vi "new.vi"(7 "waitgroups":refnum<data-value>, 8 "error in (no error)":errorcluster, 11 "max_waitgroup_processes":i32=1) -> (0 "error out":errorcluster, 3 "waitgroup":T1)   [LabVIEW 2015, in "lv-waitgroup.lvlib"]
doc: "new.vi when provided with a valid variant DVR and a set number of max_processes, it will create an ID and generate a \"Waitgroup\" reference, which combines the provided DVR reference with the ID for the waitgroup that can be used for a number of downstream/child functions. This waitgroup reference can be used to group processes under the same waitgroup. Use new.vi every time you want to group processes."
uses:
  lv-waitgroup.lvlib
  _controls/api_waitgroup.ctl
  private/_controls/waitgroup.ctl
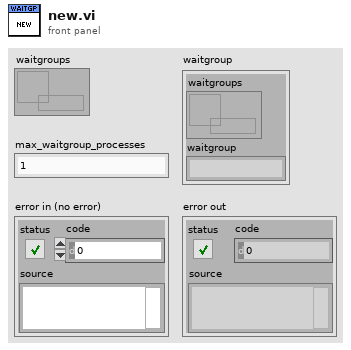
[diagram p1: front panel]
types:
  T1 = typedef "lv-waitgroup.lvlib/api_waitgroup.ctl" = cluster{"waitgroups":refnum<data-value>, "waitgroup":string}
  T2 = typedef "lv-waitgroup.lvlib/waitgroup.ctl" = cluster{"waitgroup":refnum<queue>, "queues":variant}
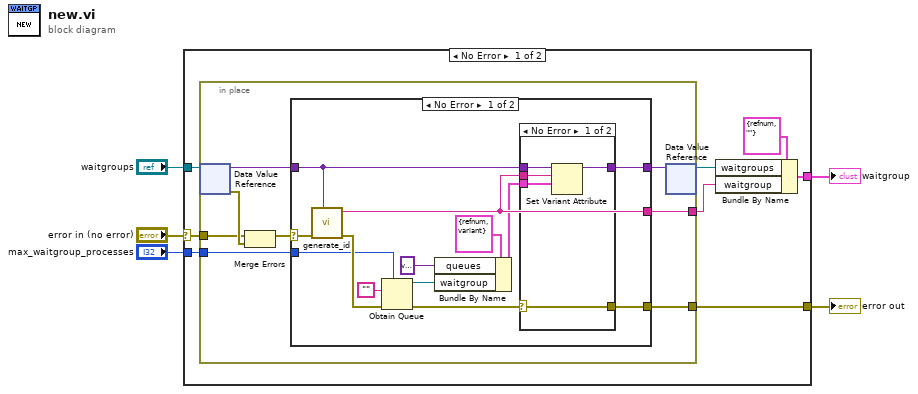
[diagram p0: block diagram]
diagram:
  n1 = case shown="No Error" "error in (no error)" {
    selector: "error in (no error)" -> [w11 w44]
    tunnel: "max_waitgroup_processes" -> [w13 _]
    tunnel: [w12 w44] -> w4
    tunnel: "waitgroups" -> [w10 _]
    tunnel: [w6 _] -> w1
    frame No Error {
      n2 = in-place {
        in-place-border: w13 -> [w19]
        in-place-border: [w14] -> w12
        in-place-border: w11 -> [w16]
        in-place-border: [w15] -> w7
        n3 = in-place-dvr #1(w10) -> (w21:variant, w20:errorcluster)
        n4 = Merge Errors(w16, w20) -> (w17:errorcluster)
        n5 = case shown="No Error" w17 {
          selector: w17 -> [w31 w42]
          tunnel: w21 -> [w30 w43]
          tunnel: w19 -> [w33 _]
          tunnel: [w32 w43] -> w18
          tunnel: [w29 _] -> w15
          tunnel: [w22 w42] -> w14
          frame No Error {
            n6 = call "generate_id.vi"("queues"=w30, "error in (no error)"=w31) -> ("error out"=w34:errorcluster, "id"=w29:string)  [unwired: 8 in]
            n7 = Obtain Queue(max queue size (-1, unlimited)=w33, element data type="", error in (no error)=w34) -> (queue out=w26:refnum<queue>, error out=w23:errorcluster)  [unwired: 2 in, 1 out]
            n8 = Bundle By Name(cluster=T2 {"waitgroup"=refnum, "queues"=variant} ("shared_data"), "queues"=variant, "waitgroup"=w26) -> (w27:T2)
            n9 = case shown="No Error" w23 {
              selector: w23 -> [w35 w41]
              tunnel: [w39 w40] -> w32
              tunnel: w30 -> [w38 w40]
              tunnel: w29 -> [w37 _]
              tunnel: w27 -> [w36 _]
              tunnel: [w35 w41] -> w22
              frame No Error {
                n10 = Set Variant Attribute(Variant=w38, name=w37, value=w36) -> (Variant out=w39:variant)  [unwired: 1 in, 2 out]
              }
              frame Error {
              }
            }
          }
          frame Error {
          }
        }
        n11 = in-place-dvr #1(w18) -> (w8:refnum<data-value>)  [unwired: 1 out]
      }
      n12 = Bundle By Name(cluster=T1 {"waitgroups"=refnum, "waitgroup"=""} ("waitgroup"), "waitgroups"=w8, "waitgroup"=w7) -> (w6:T1)
    }
    frame Error {
    }
  }
  "error out" <- w4
  "waitgroup" <- w1
